vi "worldFrame.vi"() -> (0 "引用输出":refnum<vi>)   [LabVIEW 2012]
uses:
  <vilib>/picture/3D Picture Control/NI_3D Picture Control.lvlib
panel:
  out "三维图片 2":refnum<vi>(3d-picture)
  in  "停止 2":bool
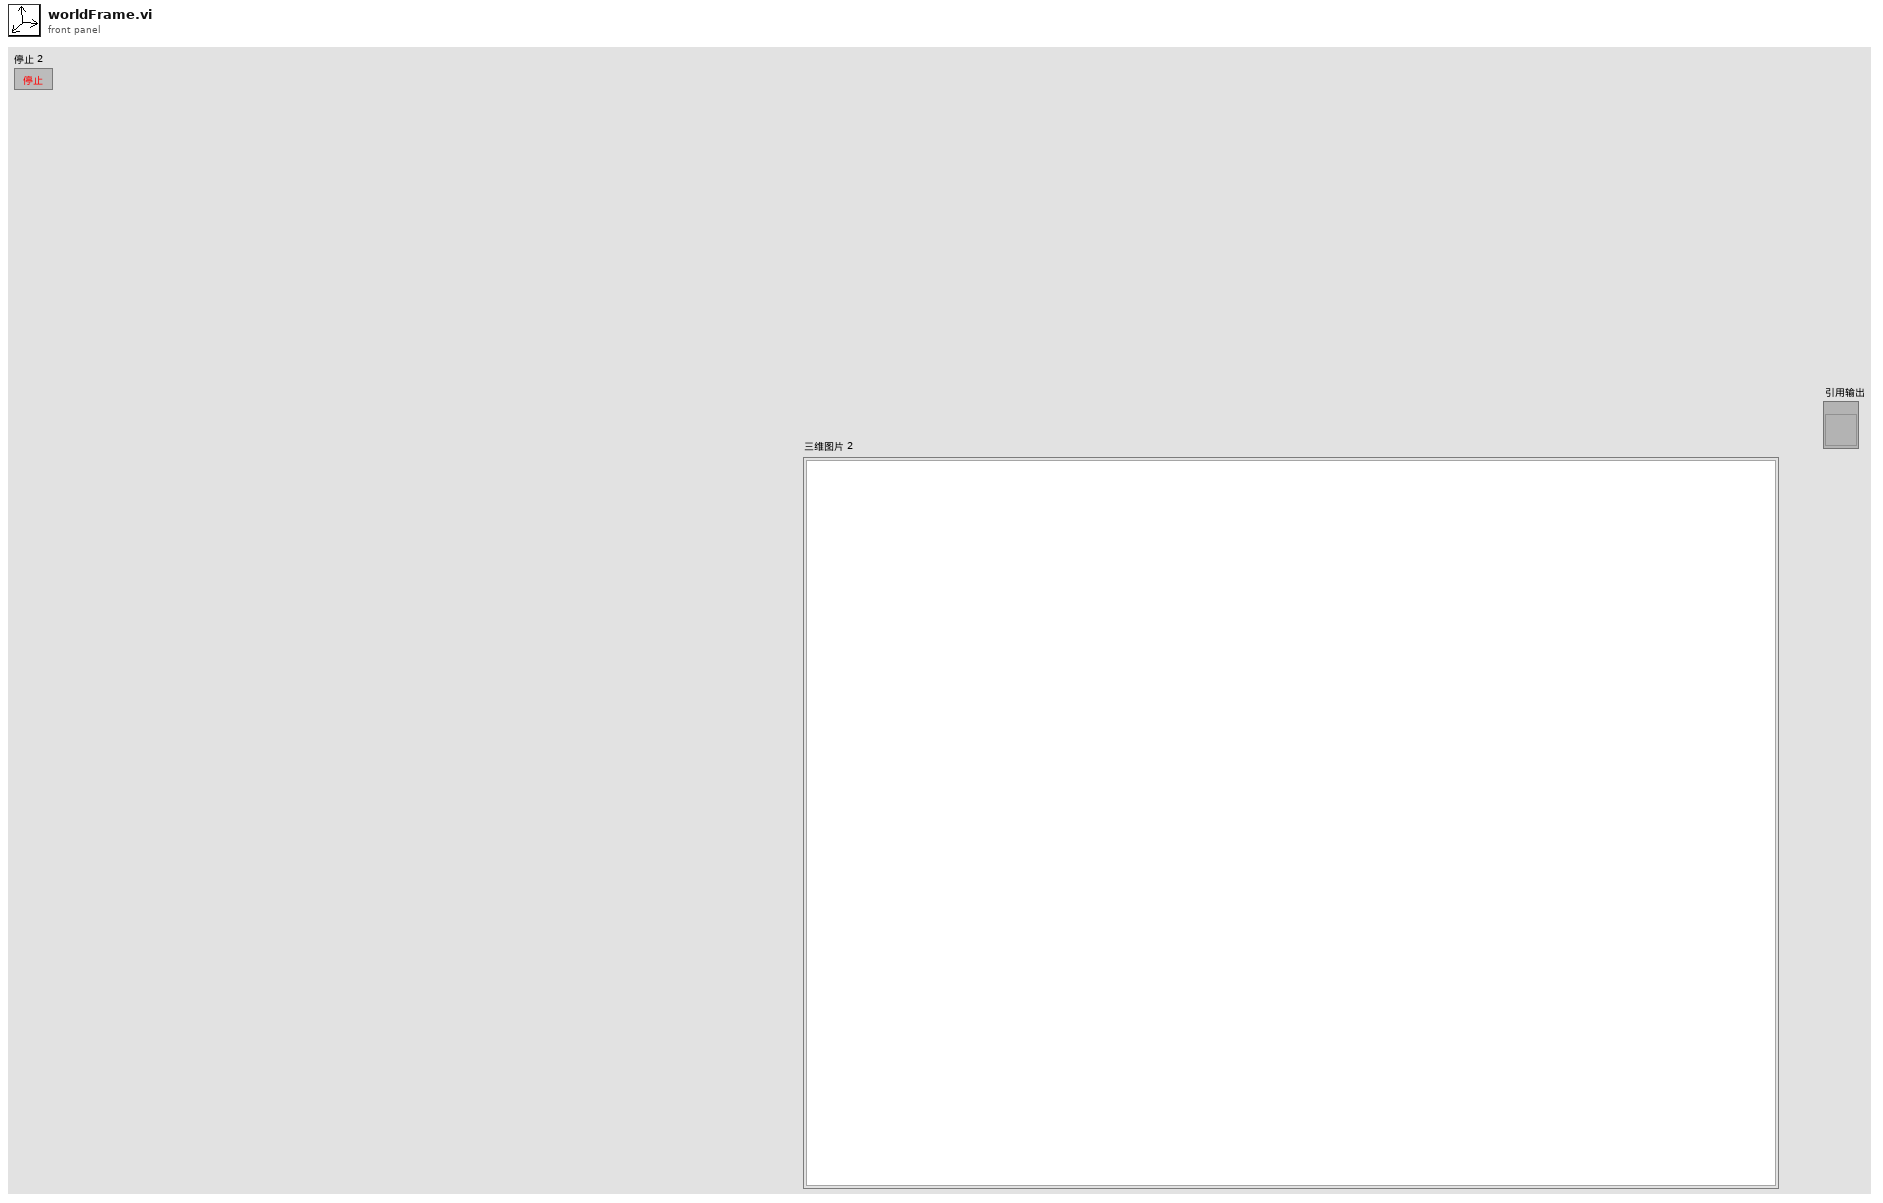
[diagram p1: front panel]
types:
  T1 = cluster{"Red":sgl, "Green":sgl, "Blue":sgl, "Alpha":sgl}
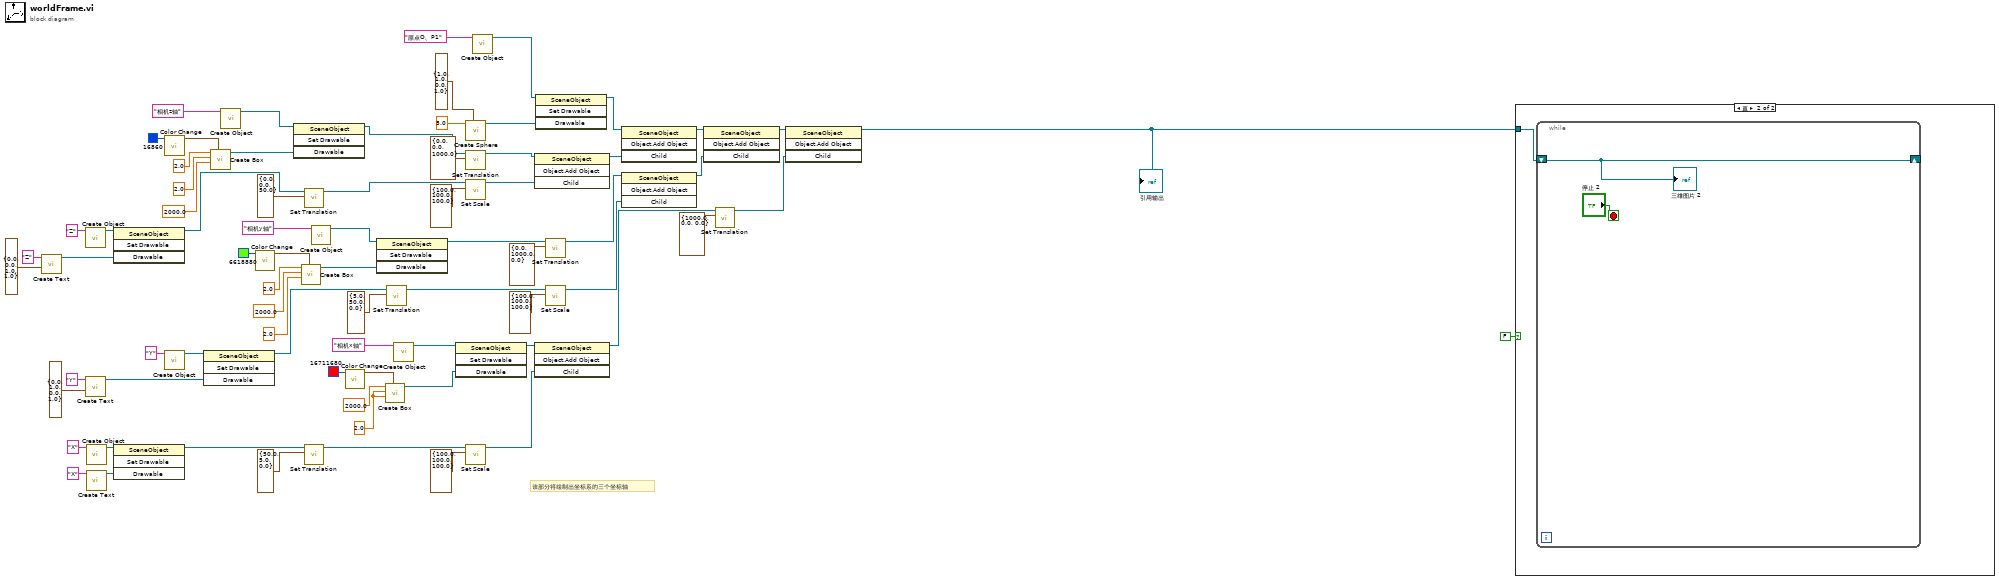
[diagram p0: block diagram]
diagram:
  w1 = sgl 2.0 ("Length Y")
  # "该部分将绘制出坐标系的三个坐标轴"
  n1 = call <vilib>:"Create Text.vi"("Color"=T1 {"Red"=0.0, "Green"=0.0, "Blue"=1.0, "Alpha"=1.0}, "Text"="Z") -> ("New Text Refnum"=w12:refnum<vi>)  [unwired: 8 in, 1 out]
  n2 = call <vilib>:"Create Object.vi"("Name"="Z") -> ("Scene:New Object"=w13:refnum<vi>)  [unwired: 9 in, 1 out]
  n3 = call <vilib>:"Create Text.vi"("Color"=T1 {"Red"=0.0, "Green"=1.0, "Blue"=0.0, "Alpha"=1.0}, "Text"="Y") -> ("New Text Refnum"=w24:refnum<vi>)  [unwired: 8 in, 1 out]
  n4 = call <vilib>:"Create Object.vi"("Name"="X") -> ("Scene:New Object"=w38:refnum<vi>)  [unwired: 9 in, 1 out]
  n5 = call <vilib>:"Create Text.vi"("Text"="X") -> ("New Text Refnum"=w37:refnum<vi>)  [unwired: 9 in, 1 out]
  n6 = invoke class="SceneObject" method="Set Drawable"(reference=w13, "Drawable"=w12) -> (reference out=w11:refnum<vi>)  [unwired: 2 in, 3 out]
  n7 = invoke class="SceneObject" method="Set Drawable"(reference=w38, "Drawable"=w37) -> (reference out=w33:refnum<vi>)  [unwired: 2 in, 3 out]
  n8 = call <vilib>:"Color Change.vi"("Color"=u32 16860) -> ("RGBA"=w55:cluster{"R":sgl, "G":sgl, "B":sgl, "A":sgl})  [unwired: 10 in]
  n9 = call <vilib>:"Create Object.vi"("Name"="Y") -> ("Scene:New Object"=w25:refnum<vi>)  [unwired: 9 in, 1 out]
  n10 = invoke class="SceneObject" method="Set Drawable"(reference=w25, "Drawable"=w24) -> (reference out=w23:refnum<vi>)  [unwired: 2 in, 3 out]
  n11 = call <vilib>:"Create Box.vi"("Color"=w55, "Length Z"=sgl 2000.0, "Length Y"=sgl 2.0, "Length X"=sgl 2.0) -> ("New Box Refnum"=w51:refnum<vi>)  [unwired: 6 in, 1 out]
  n12 = call <vilib>:"Create Object.vi"("Name"="相机z轴") -> ("Scene:New Object"=w52:refnum<vi>)  [unwired: 9 in, 1 out]
  n13 = call <vilib>:"Color Change.vi"("Color"=u32 6618880) -> ("RGBA"=w65:cluster{"R":sgl, "G":sgl, "B":sgl, "A":sgl})  [unwired: 10 in]
  n14 = invoke class="SceneObject" method="Set Drawable"(reference=w52, "Drawable"=w51) -> (reference out=w49:refnum<vi>)  [unwired: 2 in, 3 out]
  n15 = call <vilib>:"Create Box.vi"("Color"=w65, "Length Z"=sgl 2.0, "Length Y"=sgl 2000.0, "Length X"=sgl 2.0) -> ("New Box Refnum"=w61:refnum<vi>)  [unwired: 6 in, 1 out]
  n16 = call <vilib>:"Set Translation.vi"("Translation"=cluster{"X":sgl, "Y":sgl, "Z":sgl} {"X"=0.0, "Y"=0.0, "Z"=50.0}, "Scene Object"=w11) -> ("Translated Object"=w9:refnum<vi>)  [unwired: 8 in, 1 out]
  n17 = call <vilib>:"Set Translation.vi"("Translation"=cluster{"X":sgl, "Y":sgl, "Z":sgl} {"X"=50.0, "Y"=5.0, "Z"=0.0}, "Scene Object"=w33) -> ("Translated Object"=w31:refnum<vi>)  [unwired: 8 in, 1 out]
  n18 = call <vilib>:"Create Object.vi"("Name"="相机y轴") -> ("Scene:New Object"=w62:refnum<vi>)  [unwired: 9 in, 1 out]
  n19 = call <vilib>:"Color Change.vi"("Color"=u32 16711680) -> ("RGBA"=w28:cluster{"R":sgl, "G":sgl, "B":sgl, "A":sgl})  [unwired: 10 in]
  n20 = invoke class="SceneObject" method="Set Drawable"(reference=w62, "Drawable"=w61) -> (reference out=w59:refnum<vi>)  [unwired: 2 in, 3 out]
  n21 = call <vilib>:"Create Box.vi"("Color"=w28, "Length Z"=w1, "Length Y"=w1, "Length X"=sgl 2000.0) -> ("New Box Refnum"=w70:refnum<vi>)  [unwired: 6 in, 1 out]
  n22 = call <vilib>:"Set Translation.vi"("Translation"=cluster{"X":sgl, "Y":sgl, "Z":sgl} {"X"=5.0, "Y"=50.0, "Z"=0.0}, "Scene Object"=w23) -> ("Translated Object"=w21:refnum<vi>)  [unwired: 8 in, 1 out]
  n23 = call <vilib>:"Create Object.vi"("Name"="相机x轴") -> ("Scene:New Object"=w71:refnum<vi>)  [unwired: 9 in, 1 out]
  n24 = invoke class="SceneObject" method="Set Drawable"(reference=w71, "Drawable"=w70) -> (reference out=w36:refnum<vi>)  [unwired: 2 in, 3 out]
  n25 = call <vilib>:"Create Sphere.vi"("Color"=T1 {"Red"=1.0, "Green"=1.0, "Blue"=0.0, "Alpha"=1.0}, "Radius"=sgl 5.0 ("Length X")) -> ("New Sphere Refnum"=w48:refnum<vi>)  [unwired: 8 in, 1 out]
  n26 = call <vilib>:"Set Translation.vi"("Translation"=cluster{"X":sgl, "Y":sgl, "Z":sgl} {"X"=0.0, "Y"=0.0, "Z"=1000.0}, "Scene Object"=w49) -> ("Translated Object"=w5:refnum<vi>)  [unwired: 8 in, 1 out]
  n27 = call <vilib>:"Set Scale.vi"("Scale"=cluster{"X":sgl, "Y":sgl, "Z":sgl} {"X"=100.0, "Y"=100.0, "Z"=100.0}, "Scene Object"=w9) -> ("Scaled Object"=w6:refnum<vi>)  [unwired: 8 in, 1 out]
  n28 = call <vilib>:"Set Scale.vi"("Scale"=cluster{"X":sgl, "Y":sgl, "Z":sgl} {"X"=100.0, "Y"=100.0, "Z"=100.0}, "Scene Object"=w31) -> ("Scaled Object"=w30:refnum<vi>)  [unwired: 8 in, 1 out]
  n29 = call <vilib>:"Create Object.vi"("Name"="原点O、P1") -> ("Scene:New Object"=w47:refnum<vi>)  [unwired: 9 in, 1 out]
  n30 = invoke class="SceneObject" method="Object.Add Object"(reference=w5, "Child"=w6) -> (reference out=w4:refnum<vi>)  [unwired: 2 in, 3 out]
  n31 = invoke class="SceneObject" method="Object.Add Object"(reference=w36, "Child"=w30) -> (reference out=w35:refnum<vi>)  [unwired: 2 in, 3 out]
  n32 = invoke class="SceneObject" method="Set Drawable"(reference=w47, "Drawable"=w48) -> (reference out=w43:refnum<vi>)  [unwired: 2 in, 3 out]
  n33 = call <vilib>:"Set Translation.vi"("Translation"=cluster{"X":sgl, "Y":sgl, "Z":sgl} {"X"=0.0, "Y"=1000.0, "Z"=0.0}, "Scene Object"=w59) -> ("Translated Object"=w18:refnum<vi>)  [unwired: 8 in, 1 out]
  n34 = call <vilib>:"Set Scale.vi"("Scale"=cluster{"X":sgl, "Y":sgl, "Z":sgl} {"X"=100.0, "Y"=100.0, "Z"=100.0}, "Scene Object"=w21) -> ("Scaled Object"=w16:refnum<vi>)  [unwired: 8 in, 1 out]
  n35 = invoke class="SceneObject" method="Object.Add Object"(reference=w43, "Child"=w4) -> (reference out=w42:refnum<vi>)  [unwired: 2 in, 3 out]
  n36 = invoke class="SceneObject" method="Object.Add Object"(reference=w18, "Child"=w16) -> (reference out=w17:refnum<vi>)  [unwired: 2 in, 3 out]
  n37 = invoke class="SceneObject" method="Object.Add Object"(reference=w42, "Child"=w17) -> (reference out=w41:refnum<vi>)  [unwired: 2 in, 3 out]
  n38 = call <vilib>:"Set Translation.vi"("Translation"=cluster{"X":sgl, "Y":sgl, "Z":sgl} {"X"=1000.0, "Y"=0.0, "Z"=0.0}, "Scene Object"=w35) -> ("Translated Object"=w34:refnum<vi>)  [unwired: 8 in, 1 out]
  n39 = invoke class="SceneObject" method="Object.Add Object"(reference=w41, "Child"=w34) -> (reference out=w2:refnum<vi>)  [unwired: 2 in, 3 out]
  "引用输出" <- w2
  n40 = case shown="真" FALSE {
    tunnel: w2 -> [_ w75]
    frame False {
    }
    frame True {
      n41 = while {
        shift-right: [w76] -> _
        shift-left: w75 -> [w76]
        stop <- "停止 2" stop-if-true
        "三维图片 2" <- w76
      }
    }
  }
